vi "EEG信号采集及处理.vi"() -> ()   [LabVIEW 2018]
uses:
  <vilib>/Analysis/2dsp.llb/Power Spectrum (DBL).vi
  <vilib>/Instr/_visa.llb/VISA Configure Serial Port (Instr).vi
  <vilib>/Analysis/NI_AALPro.lvlib
panel:
  out "波形图":dbl[](graph)
  out "运行时间":string caption="开始时间："
  out "开始时间":string caption="开始时间："
  in  "采样周期（ms）":u32=10
  out "曲线":dbl(graph)
  in  "端口":refnum<visa-resource-name> caption="串口号"
  in  "停止按钮":bool
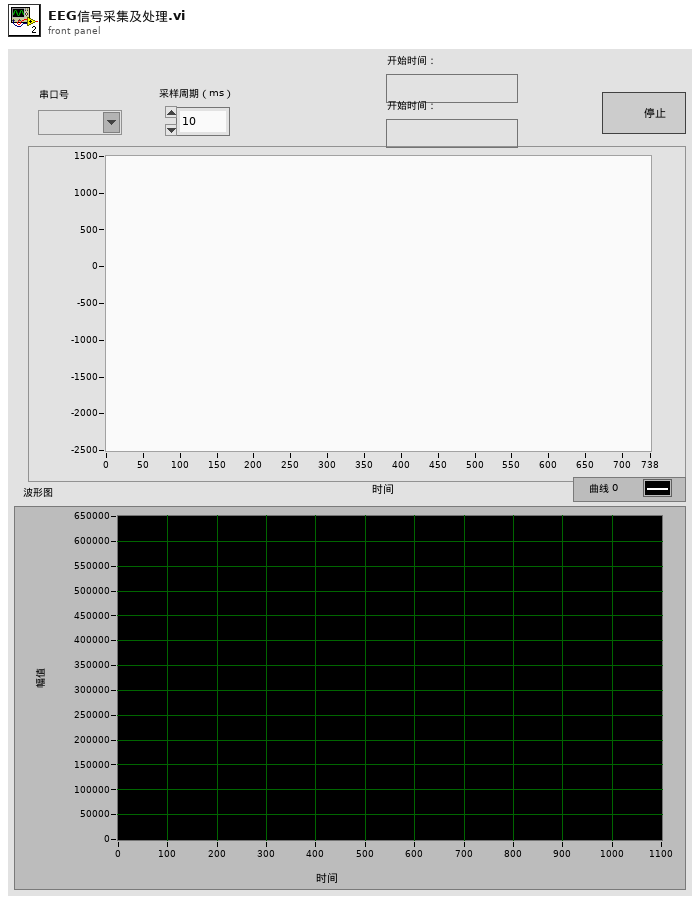
[diagram p1: front panel]
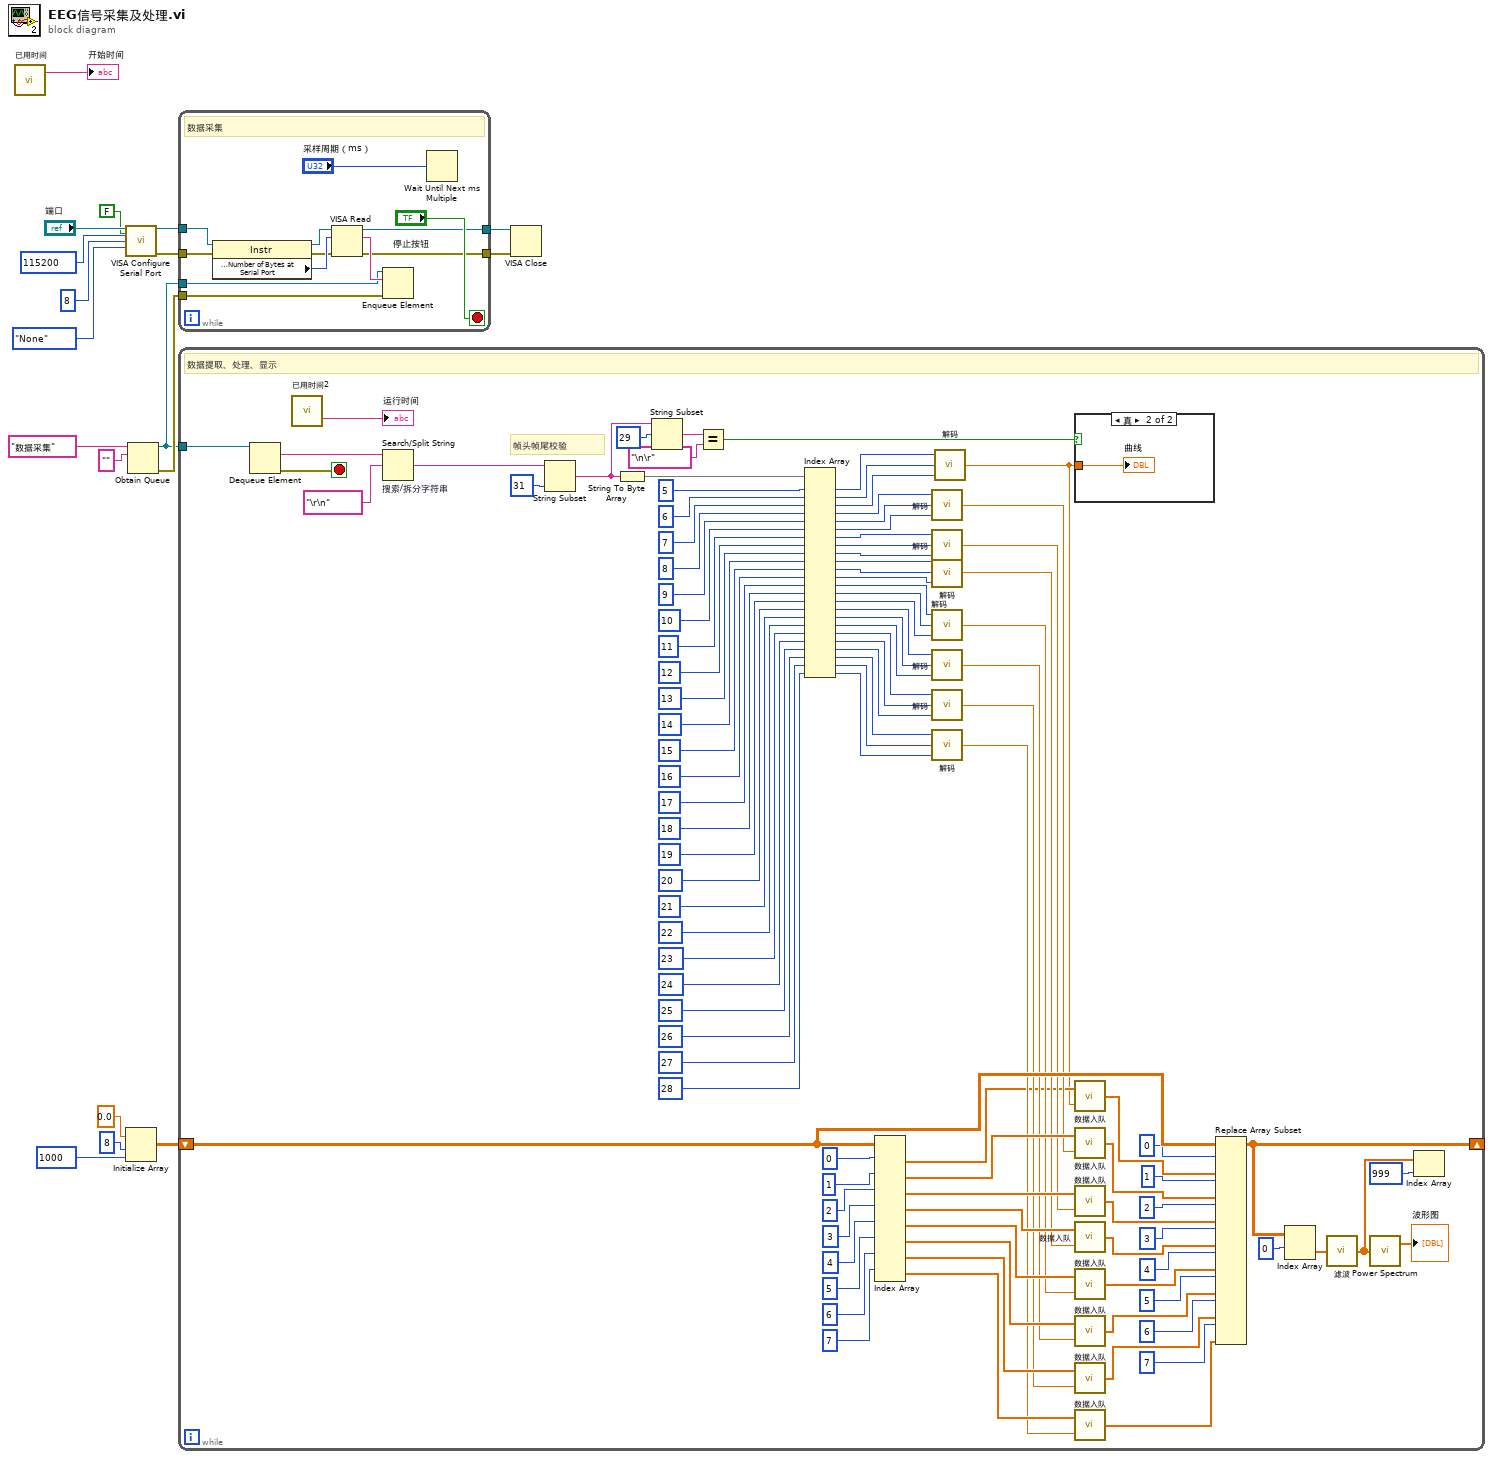
[diagram p0: block diagram]
diagram:
  n1 = call "已用时间"() -> ("Present Text"=→"开始时间":string)  [unwired: 12 in, 7 out]
  n2 = call-poly "VISA Configure Serial Port"("VISA resource name"="端口", "Enable Termination\nChar (T)"=FALSE ("Enable Termination\nChar (T)"), "baud rate (9600)"=u32 115200, "data bits (8)"=u16 8, "parity (0:none)"=enum16{"None", "Odd", "Even", "Mark", "Space"}."None") -> ("VISA resource name out"=w12:refnum<visa-resource-name>, "error out"=w7:errorcluster)  [unwired: 9 in]
  n3 = Initialize Array(0.0 ("元素"), 8 ("维数大小"), 1000 ("维数大小")) -> (w2:dbl[][])
  n4 = Obtain Queue(name (unnamed)="数据采集" ("名称（未命名）"), element data type="") -> (queue out=w5:refnum<queue>, error out=w9:errorcluster)  [unwired: 3 in, 1 out]
  n5 = while {
    tunnel: w12 -> [w28]
    tunnel: [w25] -> w10
    tunnel: w9 -> [w24]
    tunnel: w7 -> [w22]
    tunnel: [w20] -> w6
    tunnel: w5 -> [w19]
    stop <- "停止按钮" stop-if-true
    # "数据采集"
    n6 = property class="Instr"(reference=w28, error in=w22) -> (reference out=w27:refnum<visa-resource-name>, error out=w21:errorcluster, "Serial Settings:Number of Bytes at Serial Port"=w26:u32)
    n7 = VISA Read(VISA resource name=w27, byte count=w26, error in (no error)=w21) -> (VISA resource name out=w25:refnum<visa-resource-name>, read buffer=w29:string, error out=w20:errorcluster)  [unwired: 1 out]
    n8 = Enqueue Element(queue=w19, element=w29, error in (no error)=w24) -> ()  [unwired: 1 in, 3 out]
    n9 = Wait Until Next ms Multiple(millisecond multiple="采样周期（ms）") -> ()  [unwired: 1 out]
  }
  n10 = while {
    tunnel: w5 -> [w138]
    shift-right: [w111] -> _
    shift-left: w2 -> [w115]
    stop <- w123 stop-if-true
    # "帧头帧尾校验"
    # "数据提取、处理、显示"
    n11 = Dequeue Element(queue=w138) -> (element=w127:string, error out=w123:errorcluster)  [unwired: 2 in, 2 out]
    n12 = call "已用时间2"() -> ("Elapsed Time Text"=→"运行时间":string)  [unwired: 12 in, 7 out]
    n13 = Search/Split String "搜索/拆分字符串"(string=w127, search string/char (-)="\r\n" ("y")) -> (match + rest of string=w129:string)  [unwired: 1 in, 2 out]
    n14 = String Subset(string=w129, length (rest)=31 ("长度（剩余）")) -> (substring=w128:string)  [unwired: 1 in]
    n15 = String To Byte Array ("字符串至字节数组转换")(string=w128) -> (unsigned byte array=w137:u8[])
    n16 = String Subset(string=w128, offset (0)=29 ("长度（剩余）")) -> (substring=w132:string)  [unwired: 1 in]
    n17 = Equal?(x=w132, y="\n\r") -> (x = y?=w124:bool)
    n18 = Index Array(array=w137, index #1=5 ("索引"), index #2=6 ("索引 2"), index #3=7 ("索引 3"), index #4=8 ("索引"), index #5=9 ("索引"), index #6=10 ("索引"), index #7=11 ("索引"), index #8=12 ("索引"), index #9=13 ("索引"), index #10=14 ("索引"), index #11=15 ("索引"), index #12=16 ("索引"), index #13=17 ("索引"), index #14=18 ("索引"), index #15=19 ("索引"), index #16=20 ("索引"), index #17=21 ("索引"), index #18=22 ("索引"), index #19=23 ("索引"), index #20=24 ("索引"), index #21=25 ("索引"), index #22=26 ("索引"), index #23=27 ("索引"), index #24=28 ("索引")) -> (element #1=w119:u8, element #2=w118:u8, element #3=w117:u8, element #4=w82:u8, element #5=w81:u8, element #6=w80:u8, element #7=w79:u8, element #8=w78:u8, element #9=w77:u8, element #10=w76:u8, element #11=w75:u8, element #12=w74:u8, element #13=w73:u8, element #14=w72:u8, element #15=w71:u8, element #16=w70:u8, element #17=w69:u8, element #18=w68:u8, element #19=w67:u8, element #20=w66:u8, element #21=w65:u8, element #22=w64:u8, element #23=w63:u8, element #24=w62:u8)
    n19 = Index Array(array=w115, index (row) #1=0 ("索引 (行)"), index (row) #2=1 ("索引 (行)"), index (row) #3=2 ("索引 (行)"), index (row) #4=3 ("索引 (行)"), index (row) #5=4 ("索引 (行)"), index (row) #6=5 ("索引 (行)"), index (row) #7=6 ("索引 (行)"), index (row) #8=7 ("索引 (行)")) -> (element #1=w32:dbl[], element #2=w54:dbl[], element #3=w52:dbl[], element #4=w51:dbl[], element #5=w50:dbl[], element #6=w49:dbl[], element #7=w48:dbl[], element #8=w47:dbl[])  [unwired: 8 in]
    n20 = call "解码.vi"("低8位"=w80, "中8位"=w81, "高8位"=w82) -> ("输出"=w40:dbl)
    n21 = call "解码.vi"("低8位"=w77, "中8位"=w78, "高8位"=w79) -> ("输出"=w39:dbl)
    n22 = call "解码.vi"("低8位"=w74, "中8位"=w75, "高8位"=w76) -> ("输出"=w38:dbl)
    n23 = call "解码.vi"("低8位"=w71, "中8位"=w72, "高8位"=w73) -> ("输出"=w37:dbl)
    n24 = call "解码.vi"("低8位"=w68, "中8位"=w69, "高8位"=w70) -> ("输出"=w36:dbl)
    n25 = call "解码.vi"("低8位"=w65, "中8位"=w66, "高8位"=w67) -> ("输出"=w35:dbl)
    n26 = call "解码.vi"("低8位"=w62, "中8位"=w63, "高8位"=w64) -> ("输出"=w34:dbl)
    n27 = call "解码.vi"("低8位"=w117, "中8位"=w118, "高8位"=w119) -> ("输出"=w31:dbl)
    n28 = case shown="真" w124 {
      tunnel: w31 -> [_ w139]
      frame False {
      }
      frame True {
        "曲线" <- w139
      }
    }
    n29 = call "数据入队.vi"("新元素/子数组"=w31, "源数组"=w32) -> ("已删除元素的数组子集"=w33:dbl[])
    n30 = call "数据入队.vi"("新元素/子数组"=w40, "源数组"=w54) -> ("已删除元素的数组子集"=w53:dbl[])
    n31 = call "数据入队.vi"("新元素/子数组"=w39, "源数组"=w52) -> ("已删除元素的数组子集"=w46:dbl[])
    n32 = call "数据入队.vi"("新元素/子数组"=w38, "源数组"=w51) -> ("已删除元素的数组子集"=w45:dbl[])
    n33 = call "数据入队.vi"("新元素/子数组"=w37, "源数组"=w50) -> ("已删除元素的数组子集"=w44:dbl[])
    n34 = call "数据入队.vi"("新元素/子数组"=w36, "源数组"=w49) -> ("已删除元素的数组子集"=w43:dbl[])
    n35 = call "数据入队.vi"("新元素/子数组"=w35, "源数组"=w48) -> ("已删除元素的数组子集"=w42:dbl[])
    n36 = call "数据入队.vi"("新元素/子数组"=w34, "源数组"=w47) -> ("已删除元素的数组子集"=w41:dbl[])
    n37 = Replace Array Subset(array=w115, new element #1=w33, index (row) #1=0 ("禁用的索引 (行)"), new element #2=w53, index (row) #2=1 ("索引 (行)"), new element #3=w46, index (row) #3=2 ("索引 (行)"), new element #4=w45, index (row) #4=3 ("索引 (行)"), new element #5=w44, index (row) #5=4 ("索引 (行)"), new element #6=w43, index (row) #6=5 ("索引 (行)"), new element #7=w42, index (row) #7=6 ("索引 (行)"), new element #8=w41, index (row) #8=7 ("索引 (行)")) -> (w111:dbl[][])  [unwired: 8 in]
    n38 = Index Array(array=w111, index (row)=0 ("索引 (行)")) -> (element=w113:dbl[])  [unwired: 1 in]
    n39 = call "滤波.vi"("X"=w113) -> ("Filtered X"=w120:dbl[])
    n40 = call-poly <vilib>:"Power Spectrum.vi"("X"=w120) -> ("Power Spectrum"=→"波形图":dbl[])  [unwired: 1 out]
    n41 = Index Array(array=w120, index=999 ("索引")) -> ()  [unwired: 1 out]
  }
  n42 = VISA Close(VISA resource name=w10, error in (no error)=w6) -> ()  [unwired: 1 out]
